vi "Encode packed int32.vi"(7 "Field Number":i32, 10 "int32":i32[](array[numeric]), 11 "Buffer in":u8[](array[numeric]) format="%.0x") -> (3 "Buffer":u8[](array[numeric]) format="%.0x")   [LabVIEW 2020, in "LV-Proto.lvlib"]
uses:
  LV-Proto.lvlib
  Wire Type.ctl
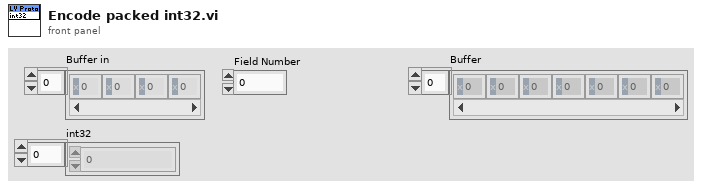
[diagram p1: front panel]
types:
  T1 = typedef "LV-Proto.lvlib/Wire Type.ctl" = enum8{"VARINT", "I64", "LEN", "SGROUP (Deprecated)", "EGROUP (Deprecated)", "I32"}
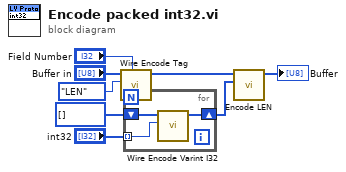
[diagram p0: block diagram]
diagram:
  n1 = call "Wire Encode Tag.vi"("Field Number"="Field Number", "Wire Type"=Wire_Type."LEN", "Buffer in"="Buffer in") -> ("Buffer"=w5:u8[])  [unwired: 8 in]
  n2 = for {
    shift-right: [w9] -> w1
    shift-left: u8[] [] ("Buffer") -> [w11]
    tunnel: "int32" -> [w10] mode=indexing
    n3 = call "Wire Encode Varint I32.vi"("I32"=w10, "Buffer in"=w11) -> ("Buffer"=w9:u8[])  [unwired: 9 in]
  }
  n4 = call "Encode LEN.vi"("Data"=w1, "Buffer in"=w5) -> ("Buffer"=→"Buffer":u8[])  [unwired: 9 in]
